vi "AlliGator Compute Phasor Plot Parameter Array.vi"(4 "Time Series Timestamps":dbl[](array[numeric]), 6 "Phasor Frequency":dbl[unit], 8 "error in (no error)":errorcluster, 9 "Parameter":T12=enum."Phasor g", 10 "Phasor Plot":T13, 11 "Raw Phasor Plot":T1 {"[Decay Metadata]"."# Folds" min=1; "[Decay Metadata]"."ROI Descriptor"."Contours"."Type" items=["No Selection", "Point", "Line", "Rectangle", "Oval", "Polygon", "Freehand Region", "Annulus", "Unused2", "Unused3", "Broken Line", "Freehand Line", "Rotated Rectangle"]}) -> (0 "error out":errorcluster, 3 "Parameter Array":dbl[](array[numeric]))   [LabVIEW 2021, in "AlliGator Phasor Graph.lvlib"]
doc: "Computes selected parameter for the phasors in a Phasor Plot of the Phasor Graph."
uses:
  AlliGator Phasor Graph.lvlib
  Graphs/XY Graph/XY Plot Data.ctl
  AlliGator Phasor Graph Parameter List.ctl
  AlliGator Raw Phasor Plot Data v4.ctl
  Phasor/Phasor (g, s).ctl
  AlliGator Decay Metadata v3.ctl
  AlliGator Decay Background Subtraction Info.ctl
  AlliGator Baseline Subtraction Method.ctl
  Graphs/XY Graph/XY Graph Plot Shift Parameters.ctl
  Graphs/XY Graph/XY Graph Plot Shift Method.ctl
  AlliGator Decay Extrapolation Parameters.ctl
  Phasor/Phasor Standard Deviation Options.ctl
  Phasor/Calibration Phasor (m, phi).ctl
  <userlib>/_OpenG.lib/array/array.llb/Filter 1D Array with Scalar (DBL)__ogtk.vi
  <userlib>/_OpenG.lib/array/array.llb/Delete Elements from 1D Array (Variant)__ogtk.vi
  <userlib>/_OpenG.lib/array/array.llb/Delete Elements from 1D Array (DBL)__ogtk.vi
  Phasor/Phasor.lvlib
  Image/Image.lvlib
  AlliGator Phasor Ratio.lvlib
  <userlib>/_OpenG.lib/array/array.llb/openg_array.lvlib
  Graphs/XY Graph/XY Graph Add-Ons.lvlib
  AlliGator Decay Preprocessing.lvlib
panel:
  # "see the AlliGator License on the block diagram (Ctrl+E or Window:Show Block Diagram)"
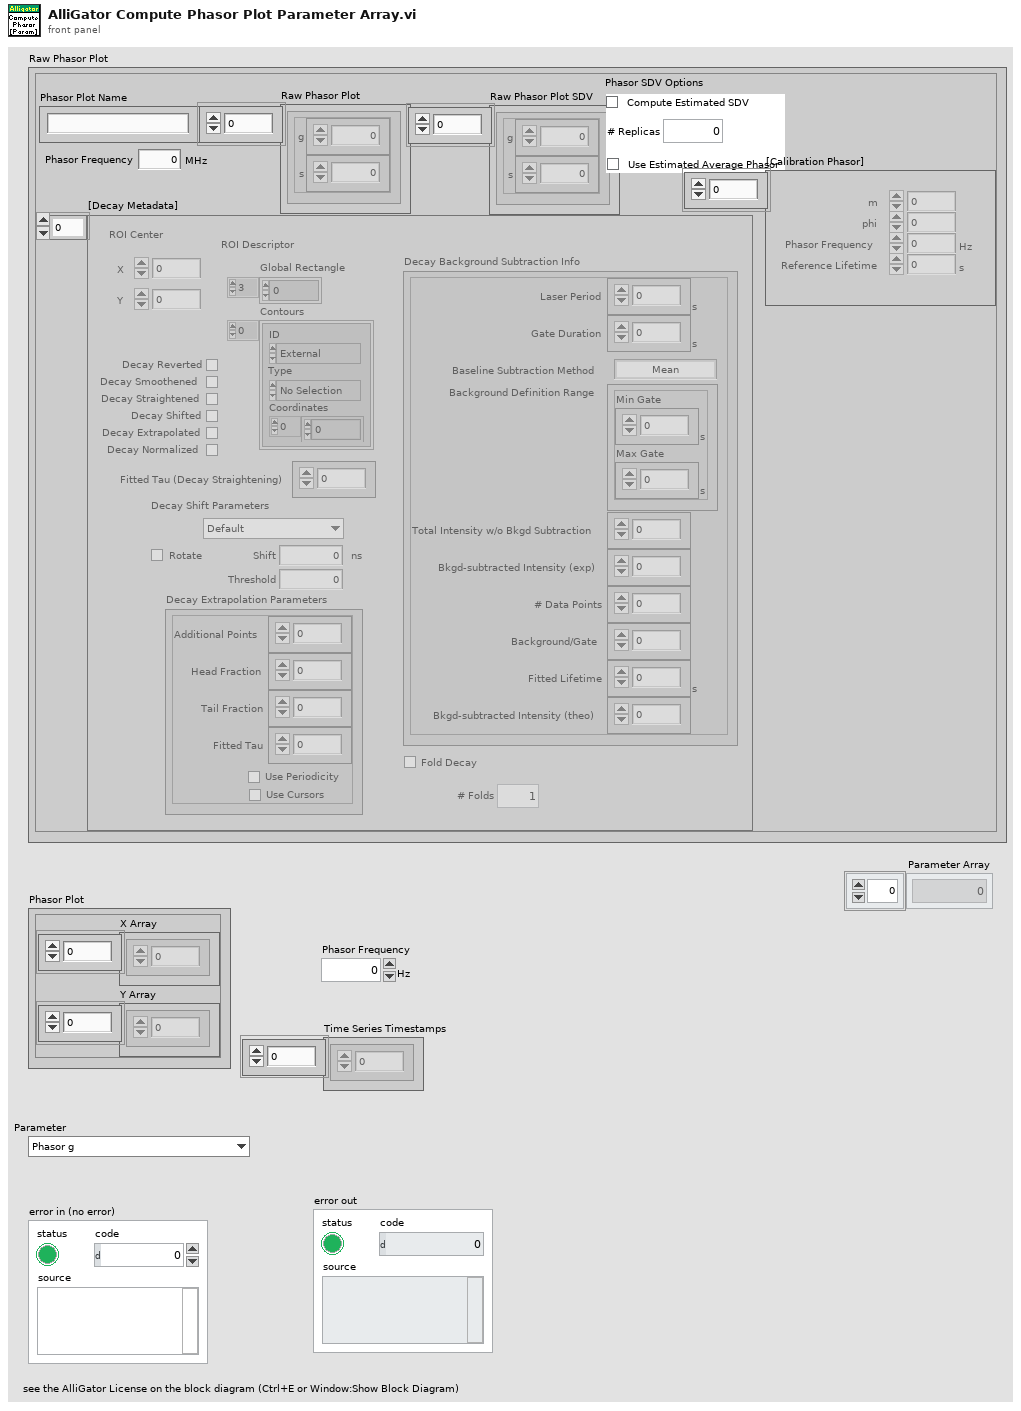
[diagram p1: front panel]
types:
  T1 = typedef "AlliGator Phasor Graph.lvlib/AlliGator Raw Phasor Plot Data v4.ctl" = cluster{"Phasor Plot Name":string, "Raw Phasor Plot":T2[], "Phasor Frequency":dbl[unit], "[Decay Metadata]":T3[], "Raw Phasor Plot SDV":T2[], "Phasor SDV Options":T10, "[Calibration Phasor]":T11[]}
  T2 = typedef "Phasor.lvlib/Phasor (g, s).ctl" = cluster{"g":dbl, "s":dbl}
  T3 = typedef "AlliGator Phasor Graph.lvlib/AlliGator Decay Metadata v3.ctl" = cluster{"ROI Descriptor":T4, "ROI Center":cluster{"X":i32, "Y":i32}, "Decay Background Subtraction Info":T5, "Decay Reverted":bool, "Decay Smoothened":bool, "Decay Straightened":bool, "Fitted Tau (Decay Straightening)":dbl, "Decay Shift Parameters":T7, "Decay Shifted":bool, "Decay Extrapolated":bool, "Decay Extrapolation Parameters":T9, "Decay Normalized":bool, "Fold Decay":bool, "# Folds":u32}
  T4 = typedef "ROI Descriptor" = cluster{"Global Rectangle":i32[], "Contours":cluster{"ID":enum32{"External", "Internal"}, "Type":u32, "Coordinates":i32[]}[]}
  T5 = typedef "AlliGator Decay Analysis.lvlib/AlliGator Decay Preprocessing.lvlib/AlliGator Decay Background Subtraction Info.ctl" = cluster{"Laser Period":dbl[unit], "Gate Duration":dbl[unit], "Baseline Subtraction Method":T6, "Background Definition Range":cluster{"Min Gate":dbl[unit], "Max Gate":dbl[unit]}, "Total Intensity w/o Bkgd Subtraction":dbl, "Bkgd-subtracted Intensity (exp)":dbl, "# Data Points":i32, "Background/Gate":dbl, "Fitted Lifetime":dbl[unit], "Bkgd-subtracted Intensity (theo)":dbl}
  T6 = typedef "AlliGator Decay Analysis.lvlib/AlliGator Decay Preprocessing.lvlib/AlliGator Baseline Subtraction Method.ctl" = enum16{"Mean", "Min", "Square Gated Single-Exponential", "File", "Constant"}
  T7 = typedef "XY Graph Add-Ons.lvlib/XY Graph Plot Shift Parameters.ctl" = cluster{"Type":T8, "Shift":dbl[unit], "Threshold":dbl, "Rotate":bool}
  T8 = typedef "XY Graph Add-Ons.lvlib/XY Graph Plot Shift Method.ctl" = enum16{"Default", "CFD", "Threshold", "Cross-Correlation"}
  T9 = typedef "AlliGator Decay Analysis.lvlib/AlliGator Decay Preprocessing.lvlib/AlliGator Decay Extrapolation Parameters.ctl" = cluster{"Additional Points":u32, "Head Fraction":dbl, "Fitted Tau":dbl, "Use Periodicity":bool, "Use Cursors":bool, "Tail Fraction":dbl}
  T10 = typedef "Phasor.lvlib/Phasor Standard Deviation Options.ctl" = cluster{"Compute Estimated SDV":bool, "# Replicas":u32, "Use Estimated Average Phasor":bool}
  T11 = typedef "Phasor.lvlib/Calibration Phasor (m, phi).ctl" = cluster{"m":dbl, "phi":dbl, "Phasor Frequency":dbl[unit], "Reference Lifetime":dbl[unit]}
  T12 = typedef "AlliGator Phasor Graph.lvlib/AlliGator Phasor Graph Parameter List.ctl" = enum16{"Time Stamp", "Index", "Phasor Parameters", "Phasor g", "Phasor s", "Phasor phi", "Phasor m", "Modulus Lifetime", "Phase Lifetime", "ROI Parameters", "ROI Center x", "ROI Center y", "ROI # pixels ", "Decay Parameters", "Intensity", "Background/Gate", "Intensity - Background", "Fitted Lifetime", "Fitted Intensity", "Phasor Ratio Parameters", "Amplitude Phasor Ratio", "Intensity Phasor Ratio", "Amplitude-Averaged Lifetime", "Intensity-Averaged Lifetime", "-", "Phasor Parameters SDV", "Phasor g SDV", "Phasor s SDV", "Phasor phi SDV", "Phasor m SDV", "Phase Lifetime SDV", "Modulus Lifetime SDV", "Phasor Ratio Parameters SDV", "Amplitude Phasor Ratio SDV", "Intensity Phasor Ratio SDV", "Amplitude-Averaged Lifetime SDV", "Intensity-Averaged Lifetime SDV"}
  T13 = typedef "XY Graph Add-Ons.lvlib/XY Plot Data.ctl" = cluster{"X Array":dbl[], "Y Array":dbl[]}
  T14 = typedef "Phasor.lvlib/Phasor (m, phi).ctl" = cluster{"m":dbl, "phi":dbl}
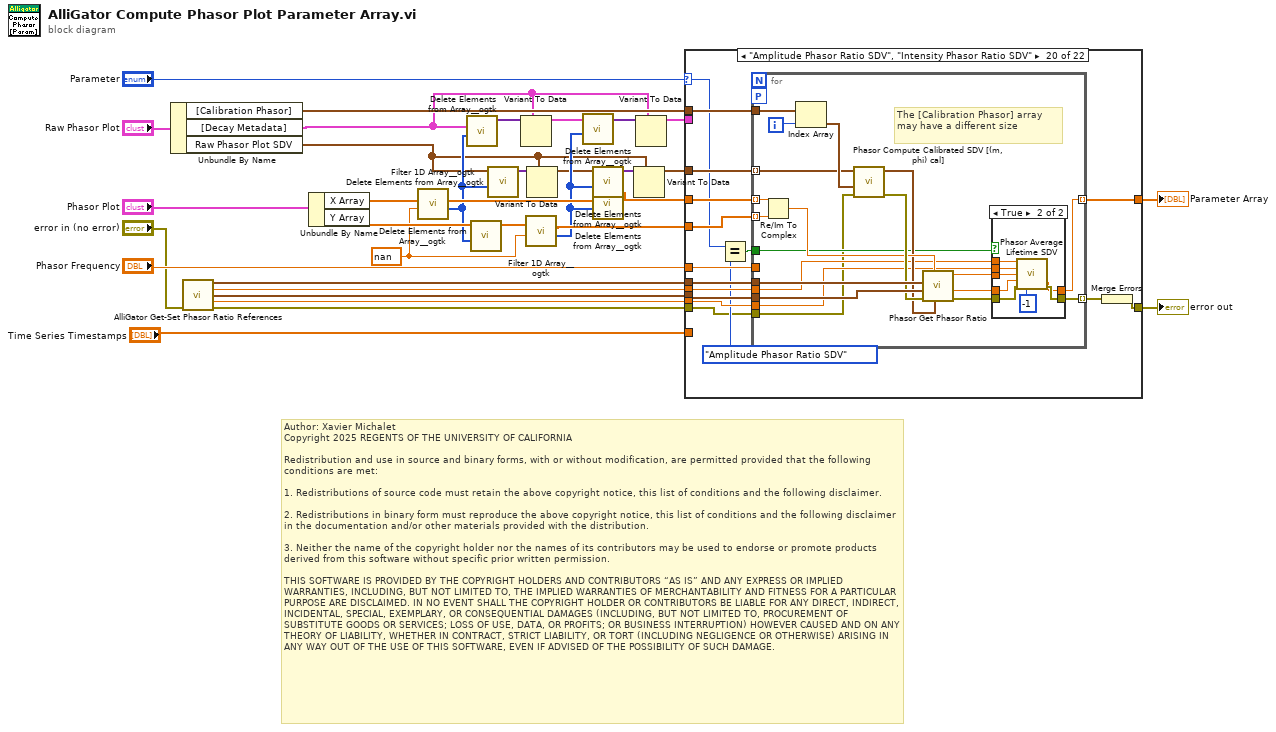
[diagram p0: block diagram]
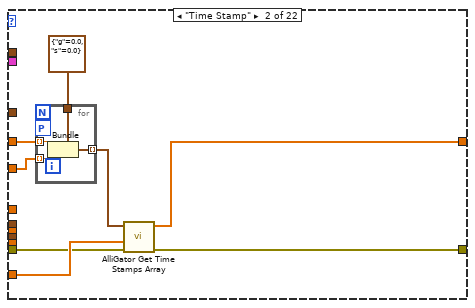
[diagram p3: hidden frame]
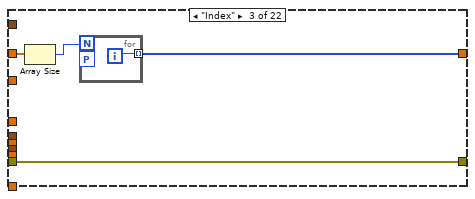
[diagram p4: hidden frame]
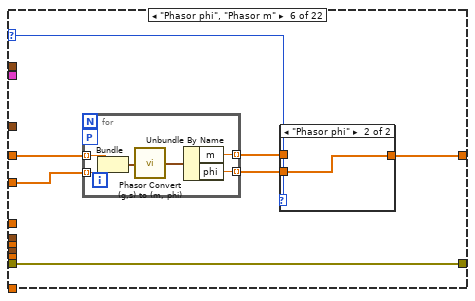
[diagram p7: hidden frame]
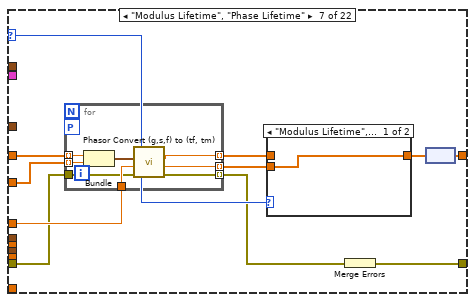
[diagram p9: hidden frame]
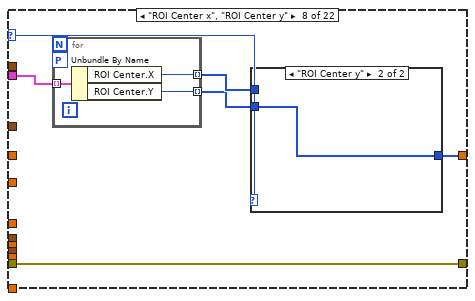
[diagram p11: hidden frame]
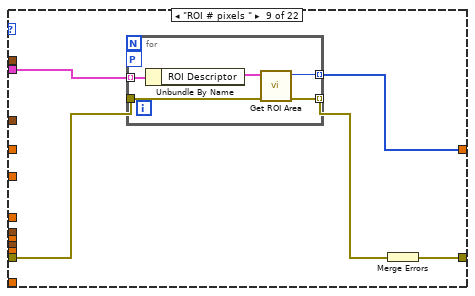
[diagram p13: hidden frame]
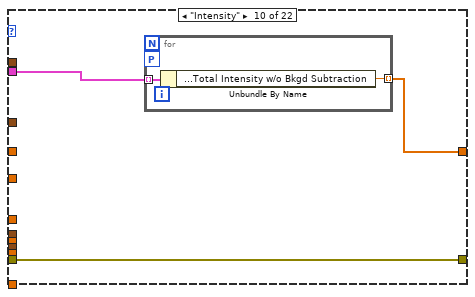
[diagram p14: hidden frame]
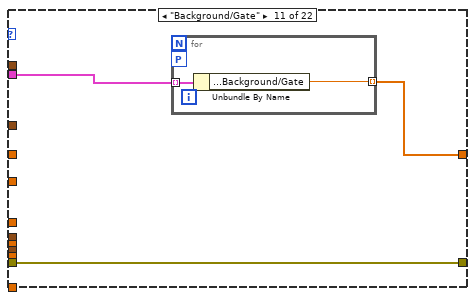
[diagram p15: hidden frame]
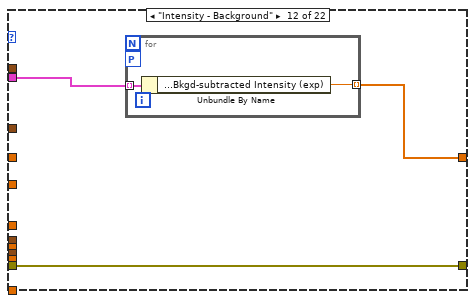
[diagram p16: hidden frame]
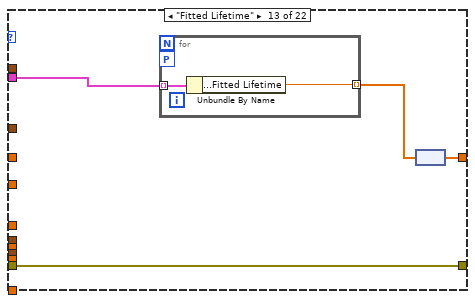
[diagram p17: hidden frame]
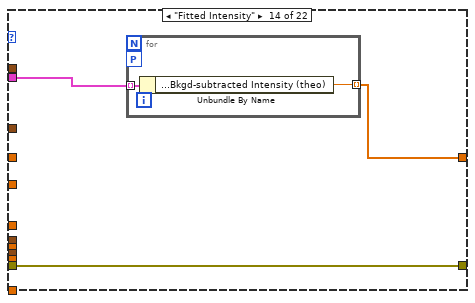
[diagram p18: hidden frame]
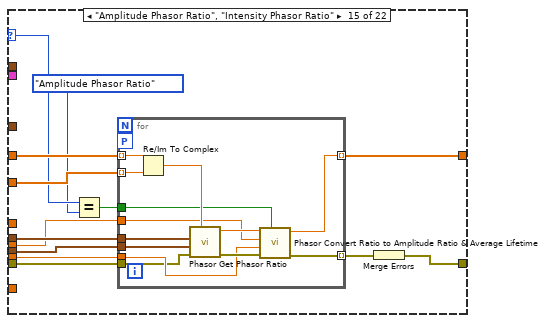
[diagram p19: hidden frame]
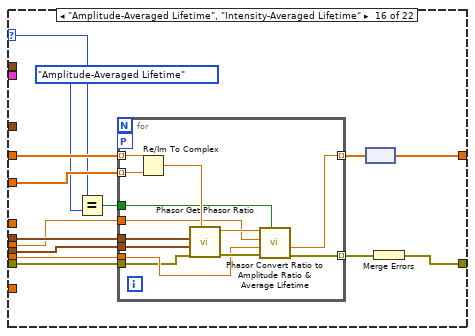
[diagram p20: hidden frame]
diagram:
  w14 = nan ("Numeric Control")
  # "Author: Xavier Michalet\nCopyright 2025 REGENTS OF THE UNIVERSITY OF CALIFORNIA\n\nRedistribution and use in source and binary forms, with or without modification, are permitted provided that the following conditions are met:\n\n1. Redistributions of source code must retain the above copyright notice, this list of conditions and the following disclaimer.\n\n2. Redistributions in binary form must reproduce the above copyright notice, this list of conditions and the following disclaimer in the documentation and/or other materials provided with the distribution.\n\n3. Neither the name of the copyright holder nor the names of its contributors may be used to endorse or promote products derived from this software without specific prior written permission.\n\nTHIS SOFTWARE IS PROVIDED BY THE COPYRIGHT HOLDERS AND CONTRIBUTORS “AS IS” AND ANY EXPRESS OR IMPLIED WARRANTIES, INCLUDING, BUT NOT LIMITED TO, THE IMPLIED WARRANTIES OF MERCHANTABILITY AND FITNESS FOR A PARTICULAR PURPOSE ARE DISCLAIMED. IN NO EVENT SHALL THE COPYRIGHT HOLDER OR CONTRIBUTORS BE LIABLE FOR ANY DIRECT, INDIRECT, INCIDENTAL, SPECIAL, EXEMPLARY, OR CONSEQUENTIAL DAMAGES (INCLUDING, BUT NOT LIMITED TO, PROCUREMENT OF SUBSTITUTE GOODS OR SERVICES; LOSS OF USE, DATA, OR PROFITS; OR BUSINESS INTERRUPTION) HOWEVER CAUSED AND ON ANY THEORY OF LIABILITY, WHETHER IN CONTRACT, STRICT LIABILITY, OR TORT (INCLUDING NEGLIGENCE OR OTHERWISE) ARISING IN ANY WAY OUT OF THE USE OF THIS SOFTWARE, EVEN IF ADVISED OF THE POSSIBILITY OF SUCH DAMAGE."
  n1 = Unbundle By Name("Raw Phasor Plot") -> ("[Calibration Phasor]"=w27:T11[], "[Decay Metadata]"=w4:T3[], "Raw Phasor Plot SDV"=w1:T2[])
  n2 = call "AlliGator Get-Set Phasor Ratio References.vi"("error in (no error)"="error in (no error)") -> ("Reference Phasor 1"=w30:T2, "Reference Lifetime 1"=w31:dbl[unit], "Reference Phasor 2"=w32:T2, "Reference Lifetime 2"=w33:dbl[unit], "error out"=w19:errorcluster)  [unwired: 7 in, 3 out]
  n3 = Unbundle By Name("Phasor Plot") -> ("X Array"=w29:dbl[], "Y Array"=w18:dbl[])
  n4 = call-poly <userlib>:"Filter 1D Array__ogtk.vi"("items to filter"=w14, "array"=w29) -> ("filtered item indices"=w11:i32[], "filtered array"=w13:dbl[])  [unwired: 4 in]
  n5 = call-poly <userlib>:"Delete Elements from Array__ogtk.vi"("indices"=w11, "array"=w4) -> ("array w/ subset deleted"=w16:variant[])  [unwired: 8 in, 1 out]
  n6 = call-poly <userlib>:"Delete Elements from Array__ogtk.vi"("indices"=w11, "array"=w18) -> ("array w/ subset deleted"=w17:dbl[])  [unwired: 8 in, 1 out]
  n7 = call-poly <userlib>:"Delete Elements from Array__ogtk.vi"("indices"=w11, "array"=w1) -> ("array w/ subset deleted"=w10:variant[])  [unwired: 8 in, 1 out]
  n8 = Variant To Data(type=w4, Variant=w16) -> (data=w8:T3[])  [unwired: 1 in, 1 out]
  n9 = call-poly <userlib>:"Filter 1D Array__ogtk.vi"("items to filter"=w14, "array"=w17) -> ("filtered item indices"=w9:i32[], "filtered array"=w15:dbl[])  [unwired: 4 in]
  n10 = Variant To Data(type=w1, Variant=w10) -> (data=w7:T2[])  [unwired: 1 in, 1 out]
  n11 = call-poly <userlib>:"Delete Elements from Array__ogtk.vi"("indices"=w9, "array"=w8) -> ("array w/ subset deleted"=w6:variant[])  [unwired: 8 in, 1 out]
  n12 = call-poly <userlib>:"Delete Elements from Array__ogtk.vi"("indices"=w9, "array"=w7) -> ("array w/ subset deleted"=w3:variant[])  [unwired: 8 in, 1 out]
  n13 = call-poly <userlib>:"Delete Elements from Array__ogtk.vi"("indices"=w9, "array"=w13) -> ("array w/ subset deleted"=w12:dbl[])  [unwired: 8 in, 1 out]
  n14 = Variant To Data(type=w1, Variant=w3) -> (data=w2:T2[])  [unwired: 1 in, 1 out]
  n15 = Variant To Data(type=w4, Variant=w6) -> (data=w5:T3[])  [unwired: 1 in, 1 out]
  n16 = case shown="\"Amplitude Phasor Ratio SDV\", \"Intensity Phasor Ratio SDV\"" "Parameter" {
    selector: "Parameter" -> [_ _ _ _ _ w60 w77 w97 _ _ _ _ _ _ w142 w168 w201 _ _ w263 w310 _]
    tunnel: w12 -> [_ w38 w50 w53 _ w62 w81 _ _ _ _ _ _ _ w149 w176 w196 w219 w241 w272 w319 _]
    tunnel: [_ w40 w49 w53 w55 w58 w79 w95 w107 w114 w119 w124 w129 w135 w143 w171 w199 w220 w242 w267 w307 _] -> w22
    tunnel: w15 -> [_ w37 _ _ w55 w61 w80 _ _ _ _ _ _ _ w148 w175 w195 w218 w240 w271 w318 _]
    tunnel: "Phasor Frequency" -> [_ _ _ _ _ _ w78 _ _ _ _ _ _ _ _ _ _ w221 w243 w273 w320 _]
    tunnel: w5 -> [_ _ _ _ _ _ _ w93 w106 w115 w120 w125 w131 w136 _ _ _ _ _ _ _ _]
    tunnel: w30 -> [_ _ _ _ _ _ _ _ _ _ _ _ _ _ w151 w178 _ _ _ w269 w316 _]
    tunnel: w31 -> [_ _ _ _ _ _ _ _ _ _ _ _ _ _ w146 w173 _ _ _ w265 w312 _]
    tunnel: w32 -> [_ _ _ _ _ _ _ _ _ _ _ _ _ _ w150 w177 _ _ _ w268 w315 _]
    tunnel: w33 -> [_ _ _ _ _ _ _ _ _ _ _ _ _ _ w147 w174 _ _ _ w264 w311 _]
    tunnel: w2 -> [_ _ _ _ _ _ _ _ _ _ _ _ _ _ _ _ w202 w215 w246 w275 w322 _]
    tunnel: [w34 w39 w48 w52 w54 w56 w72 w92 w103 w113 w118 w123 w128 w134 w144 w169 w193 w216 w238 w270 w317 w346] -> w25
    tunnel: w27 -> [_ _ _ _ _ _ _ _ _ _ _ _ _ _ _ _ w197 w223 w245 w274 w321 _]
    tunnel: w19 -> [w34 w41 w48 w52 w54 w56 w71 w92 w105 w113 w118 w123 w128 w134 w139 w165 w192 w214 w237 w260 w306 w346]
    tunnel: "Time Series Timestamps" -> [_ w42 _ _ _ _ _ _ _ _ _ _ _ _ _ _ _ _ _ _ _ _]
    frame "-", Default {
    }
    frame "Time Stamp" {
      n17 = for {
        tunnel: w38 -> [w46] mode=indexing
        tunnel: w37 -> [w45] mode=indexing
        tunnel: T2 {"g"=0.0, "s"=0.0} ("Phasor (g, s)") -> [w44]
        tunnel: [w43] -> w35 mode=indexing
        workers-P: _ -> [_]
        n18 = Bundle(cluster=w44, "g"=w46, "s"=w45) -> (w43:T2)
      }
      n19 = call "AlliGator Get Time Stamps Array.vi"("Error In"=w41, "Dataset Series Timestamps in"=w42, "Phasor Array"=w35) -> ("Error Out"=w39:errorcluster, "Dataset Series Timestamps out"=w40:dbl[])  [unwired: 7 in]
    }
    frame "Index" {
      n20 = Array Size(array=w50) -> (size(s)=w47:i32)
      n21 = for {
        N: w47 -> [_]
        tunnel: [w51] -> w49 mode=indexing
        workers-P: _ -> [_]
        i -> [w51]
      }
    }
    frame "Phasor g" {
    }
    frame "Phasor s" {
    }
    frame "Phasor phi", "Phasor m" {
      n22 = for {
        tunnel: w62 -> [w70] mode=indexing
        tunnel: w61 -> [w69] mode=indexing
        tunnel: [w66] -> w59 mode=indexing
        tunnel: [w65] -> w57 mode=indexing
        workers-P: _ -> [_]
        n23 = Bundle(w70, "Numeric"=w69) -> (w68:cluster{dbl, "Numeric":dbl})  [unwired: 1 in]
        n24 = call "Phasor Convert (g,s) to (m, phi).vi"("Phasor (g, s)"=w68) -> ("Phasor (m, phi)"=w67:T14)  [unwired: 8 in]
        n25 = Unbundle By Name(w67) -> ("m"=w66:dbl, "phi"=w65:dbl)
      }
      n26 = case shown="\"Phasor phi\"" w60 {
        tunnel: w59 -> [w63 _]
        tunnel: [w63 w64] -> w58
        tunnel: w57 -> [_ w64]
        frame "Phasor m", Default {
        }
        frame "Phasor phi" {
        }
      }
    }
    frame "Modulus Lifetime", "Phase Lifetime" {
      n27 = for {
        tunnel: w81 -> [w91] mode=indexing
        tunnel: w80 -> [w90] mode=indexing
        tunnel: [w88] -> w76 mode=indexing
        tunnel: [w87] -> w74 mode=indexing
        tunnel: w78 -> [w86]
        tunnel: [w85] -> w73 mode=indexing
        tunnel: w71 -> [w84]
        workers-P: _ -> [_]
        n28 = Bundle(w91, "Numeric"=w90) -> (w89:cluster{dbl, "Numeric":dbl})  [unwired: 1 in]
        n29 = call "Phasor Convert (g,s,f) to (tf, tm).vi"("Error In"=w84, "Phasor Harmonic Frequency"=w86, "Phasor (g, s)"=w89) -> ("Error Out"=w85:errorcluster, "Modulus Lifetime"=w87:dbl[unit], "Phase Lifetime"=w88:dbl[unit])  [unwired: 6 in]
      }
      n30 = case shown="\"Modulus Lifetime\", Default" w77 {
        tunnel: w76 -> [_ w83]
        tunnel: [w82 w83] -> w75
        tunnel: w74 -> [w82 _]
        frame "Modulus Lifetime", Default {
        }
        frame "Phase Lifetime" {
        }
      }
      n31 = Merge Errors(w73) -> (w72:errorcluster)
      n32 = node(w75) -> (w79:dbl[])
    }
    frame "ROI Center x", "ROI Center y" {
      n33 = for {
        tunnel: w93 -> [w102] mode=indexing
        tunnel: [w101] -> w96 mode=indexing
        tunnel: [w100] -> w94 mode=indexing
        workers-P: _ -> [_]
        n34 = Unbundle By Name(w102) -> ("ROI Center.X"=w101:i32, "ROI Center.Y"=w100:i32)
      }
      n35 = case shown="\"ROI Center y\"" w97 {
        tunnel: w96 -> [w98 _]
        tunnel: [w98 w99] -> w95
        tunnel: w94 -> [_ w99]
        frame "ROI Center x", Default {
        }
        frame "ROI Center y" {
        }
      }
    }
    frame "ROI # pixels " {
      n36 = for {
        tunnel: w106 -> [w112] mode=indexing
        tunnel: [w110] -> w107 mode=indexing
        tunnel: w105 -> [w109]
        tunnel: [w108] -> w104 mode=indexing
        workers-P: _ -> [_]
        n37 = Unbundle By Name(w112) -> ("ROI Descriptor"=w111:T4)
        n38 = call "Get ROI Area.vi"("Error In"=w109, "ROI Descriptor"=w111) -> ("Error Out"=w108:errorcluster, "Number of Pixels"=w110:u32)  [unwired: 8 in]
      }
      n39 = Merge Errors(w104) -> (w103:errorcluster)
    }
    frame "Intensity" {
      n40 = for {
        tunnel: w115 -> [w117] mode=indexing
        tunnel: [w116] -> w114 mode=indexing
        workers-P: _ -> [_]
        n41 = Unbundle By Name(w117) -> ("Decay Background Subtraction Info.Total Intensity w/o Bkgd Subtraction"=w116:dbl)
      }
    }
    frame "Background/Gate" {
      n42 = for {
        tunnel: w120 -> [w122] mode=indexing
        tunnel: [w121] -> w119 mode=indexing
        workers-P: _ -> [_]
        n43 = Unbundle By Name(w122) -> ("Decay Background Subtraction Info.Background/Gate"=w121:dbl)
      }
    }
    frame "Intensity - Background" {
      n44 = for {
        tunnel: w125 -> [w127] mode=indexing
        tunnel: [w126] -> w124 mode=indexing
        workers-P: _ -> [_]
        n45 = Unbundle By Name(w127) -> ("Decay Background Subtraction Info.Bkgd-subtracted Intensity (exp)"=w126:dbl)
      }
    }
    frame "Fitted Lifetime" {
      n46 = for {
        tunnel: w131 -> [w133] mode=indexing
        tunnel: [w132] -> w130 mode=indexing
        workers-P: _ -> [_]
        n47 = Unbundle By Name(w133) -> ("Decay Background Subtraction Info.Fitted Lifetime"=w132:dbl[unit])
      }
      n48 = node(w130) -> (w129:dbl[])
    }
    frame "Fitted Intensity" {
      n49 = for {
        tunnel: w136 -> [w138] mode=indexing
        tunnel: [w137] -> w135 mode=indexing
        workers-P: _ -> [_]
        n50 = Unbundle By Name(w138) -> ("Decay Background Subtraction Info.Bkgd-subtracted Intensity (theo)"=w137:dbl)
      }
    }
    frame "Amplitude Phasor Ratio", "Intensity Phasor Ratio" {
      n51 = Equal?(x=w142, y=AlliGator_Phasor_Graph_Parameter_List."Amplitude Phasor Ratio") -> (x = y?=w141:bool)
      n52 = for {
        tunnel: w151 -> [w164]
        tunnel: w150 -> [w163]
        tunnel: w149 -> [w162] mode=indexing
        tunnel: w148 -> [w161] mode=indexing
        tunnel: w147 -> [w157]
        tunnel: w146 -> [w156]
        tunnel: [w154] -> w143 mode=indexing
        tunnel: [w155] -> w145 mode=indexing
        tunnel: w141 -> [w153]
        tunnel: w139 -> [w152]
        workers-P: _ -> [_]
        n53 = Re/Im To Complex(1:w161, 2:w162) -> (0:w160:cdb)
        n54 = call "Phasor Get Phasor Ratio.vi"("z"=w160, "Error In"=w152, "Reference Phasor 2"=w163, "Reference Phasor 1"=w164) -> ("Error Out"=w158:errorcluster, "Phasor Ratio (f1)"=w159:dbl)  [unwired: 5 in, 1 out]
        n55 = call "Phasor Convert Ratio to Amplitude Ratio & Average Lifetime.vi"("Compute Amplitude Ratio"=w153, "error in (no error)"=w158, "Reference Lifetime 2"=w157, "Reference Lifetime 1"=w156, "Phasor Ratio (f1)"=w159) -> ("error out"=w155:errorcluster, "Phasor/Amplitude Ratio"=w154:dbl)  [unwired: 2 in, 3 out]
      }
      n56 = Merge Errors(w145) -> (w144:errorcluster)
    }
    frame "Amplitude-Averaged Lifetime", "Intensity-Averaged Lifetime" {
      n57 = Equal?(x=w168, y=AlliGator_Phasor_Graph_Parameter_List."Amplitude-Averaged Lifetime") -> (x = y?=w167:bool)
      n58 = for {
        tunnel: w178 -> [w191]
        tunnel: w177 -> [w190]
        tunnel: w176 -> [w189] mode=indexing
        tunnel: w175 -> [w188] mode=indexing
        tunnel: w174 -> [w184]
        tunnel: w173 -> [w183]
        tunnel: [w182] -> w172 mode=indexing
        tunnel: [w181] -> w170 mode=indexing
        tunnel: w167 -> [w180]
        tunnel: w165 -> [w179]
        workers-P: _ -> [_]
        n59 = Re/Im To Complex(1:w188, 2:w189) -> (0:w187:cdb)
        n60 = call "Phasor Get Phasor Ratio.vi"("z"=w187, "Error In"=w179, "Reference Phasor 2"=w190, "Reference Phasor 1"=w191) -> ("Error Out"=w185:errorcluster, "Phasor Ratio (f1)"=w186:dbl)  [unwired: 5 in, 1 out]
        n61 = call "Phasor Convert Ratio to Amplitude Ratio & Average Lifetime.vi"("Compute Amplitude Ratio"=w180, "error in (no error)"=w185, "Reference Lifetime 2"=w184, "Reference Lifetime 1"=w183, "Phasor Ratio (f1)"=w186) -> ("error out"=w181:errorcluster, "Average Lifetime"=w182:dbl[unit])  [unwired: 2 in, 3 out]
      }
      n62 = node(w172) -> (w171:dbl[])
      n63 = Merge Errors(w170) -> (w169:errorcluster)
    }
    frame "Phasor g SDV", "Phasor s SDV" {
      # "The [Calibration Phasor] array may have a different size"
      n64 = for {
        tunnel: w202 -> [w206] mode=indexing
        tunnel: [w213] -> w200 mode=indexing
        tunnel: [w212] -> w198 mode=indexing
        tunnel: w197 -> [w211]
        tunnel: w196 -> [_] mode=indexing
        tunnel: w195 -> [_] mode=indexing
        tunnel: [w207] -> w194 mode=indexing
        tunnel: w192 -> [w205]
        workers-P: _ -> [_]
        i -> [w210]
        n65 = Index Array(array=w211, index=w210) -> (element=w209:T11)
        n66 = call "Phasor Compute Calibrated SDV [(m, phi) cal].vi"("error in"=w205, "Calibration Phasor"=w209, "Raw Phasor"=w206) -> ("error out"=w207:errorcluster, "Calibrated Phasor SDV (g, s)"=w208:T2)  [unwired: 7 in]
        n67 = Unbundle By Name(w208) -> ("g"=w213:dbl, "s"=w212:dbl)
      }
      n68 = case shown="\"Phasor s\"" w201 {
        tunnel: w200 -> [w203 _]
        tunnel: [w203 w204] -> w199
        tunnel: w198 -> [_ w204]
        frame "Phasor g", Default {
        }
        frame "Phasor s" {
        }
      }
      n69 = Merge Errors(w194) -> (w193:errorcluster)
    }
    frame "Phase Lifetime SDV" {
      # "The [Calibration Phasor] array may have a different size"
      n70 = for {
        tunnel: [w234] -> w222 mode=indexing
        tunnel: w223 -> [w236]
        tunnel: w221 -> [w233]
        tunnel: w219 -> [w232] mode=indexing
        tunnel: w218 -> [w231] mode=indexing
        tunnel: [w230] -> w217 mode=indexing
        tunnel: w215 -> [w225] mode=indexing
        tunnel: w214 -> [w224]
        workers-P: _ -> [_]
        i -> [w235]
        n71 = Bundle(w232, "Numeric"=w231) -> (w226:cluster{dbl, "Numeric":dbl})  [unwired: 1 in]
        n72 = Index Array(array=w236, index=w235) -> (element=w229:T11)
        n73 = call "Phasor Compute Calibrated SDV [(m, phi) cal].vi"("error in"=w224, "Calibration Phasor"=w229, "Raw Phasor"=w225) -> ("error out"=w228:errorcluster, "Calibrated Phasor SDV (g, s)"=w227:T2)  [unwired: 7 in]
        n74 = call "Phasor Compute tau_phi SDV.vi"("Error In"=w228, "Phasor Frequency"=w233, "Phasor SDV (g, s)"=w227, "Phasor (g, s)"=w226) -> ("Error Out"=w230:errorcluster, "tau_phi SDV"=w234:dbl[unit])  [unwired: 6 in]
      }
      n75 = Merge Errors(w217) -> (w216:errorcluster)
      n76 = node(w222) -> (w220:dbl[])
    }
    frame "Modulus Lifetime SDV" {
      # "The [Calibration Phasor] array may have a different size"
      n77 = for {
        tunnel: w246 -> [w248] mode=indexing
        tunnel: [w257] -> w244 mode=indexing
        tunnel: w245 -> [w259]
        tunnel: w243 -> [w256]
        tunnel: w241 -> [w253] mode=indexing
        tunnel: w240 -> [w252] mode=indexing
        tunnel: [w251] -> w239 mode=indexing
        tunnel: w237 -> [w247]
        workers-P: _ -> [_]
        i -> [w258]
        n78 = Bundle(w253, "Numeric"=w252) -> (w250:cluster{dbl, "Numeric":dbl})  [unwired: 1 in]
        n79 = Index Array(array=w259, index=w258) -> (element=w249:T11)
        n80 = call "Phasor Compute Calibrated SDV [(m, phi) cal].vi"("error in"=w247, "Calibration Phasor"=w249, "Raw Phasor"=w248) -> ("error out"=w255:errorcluster, "Calibrated Phasor SDV (g, s)"=w254:T2)  [unwired: 7 in]
        n81 = call "Phasor Compute tau_m SDV.vi"("Error In"=w255, "Phasor Frequency"=w256, "Phasor SDV (g, s)"=w254, "Phasor (g, s)"=w250) -> ("Error Out"=w251:errorcluster, "<tau_m>"=w257:dbl[unit])  [unwired: 5 in, 1 out]
      }
      n82 = Merge Errors(w239) -> (w238:errorcluster)
      n83 = node(w244) -> (w242:dbl[])
    }
    frame "Amplitude Phasor Ratio SDV", "Intensity Phasor Ratio SDV" {
      n84 = Equal?(x=w263, y=AlliGator_Phasor_Graph_Parameter_List."Amplitude Phasor Ratio SDV") -> (x = y?=w261:bool)
      n85 = for {
        tunnel: w275 -> [w289] mode=indexing
        tunnel: w274 -> [w295]
        tunnel: w273 -> [_]
        tunnel: w272 -> [w288] mode=indexing
        tunnel: w271 -> [w287] mode=indexing
        tunnel: w269 -> [w293]
        tunnel: w268 -> [w292]
        tunnel: [w277] -> w267 mode=indexing
        tunnel: [w278] -> w266 mode=indexing
        tunnel: w265 -> [w281]
        tunnel: w264 -> [w280]
        tunnel: w261 -> [w279]
        tunnel: w260 -> [w276]
        workers-P: _ -> [_]
        i -> [w294]
        # "The [Calibration Phasor] array may have a different size"
        n86 = Re/Im To Complex(1:w287, 2:w288) -> (0:w286:cdb)
        n87 = Index Array(array=w295, index=w294) -> (element=w291:T11)
        n88 = call "Phasor Compute Calibrated SDV [(m, phi) cal].vi"("error in"=w276, "Calibration Phasor"=w291, "Raw Phasor"=w289) -> ("error out"=w290:errorcluster, "Calibrated Phasor SDV (g, s)"=w285:T2)  [unwired: 7 in]
        n89 = call "Phasor Get Phasor Ratio.vi"("Phasor SDV"=w285, "z"=w286, "Error In"=w290, "Reference Phasor 2"=w292, "Reference Phasor 1"=w293) -> ("Error Out"=w282:errorcluster, "Phasor Ratio SDV"=w283:dbl, "Phasor Ratio (f1)"=w284:dbl)  [unwired: 4 in]
        n90 = case shown="True" w279 {
          tunnel: w284 -> [_ w305]
          tunnel: w283 -> [w296 w304]
          tunnel: w282 -> [w297 w303]
          tunnel: w281 -> [_ w302]
          tunnel: w280 -> [_ w301]
          tunnel: [w297 w300] -> w278
          tunnel: [w296 w299] -> w277
          frame False {
          }
          frame True {
            n91 = call "Phasor Average Lifetime SDV.vi"("tau 1"=w302, "tau 2"=w301, "r"=w305, "SDV r"=w304, "Error In"=w303, "seed"=-1) -> ("SDV a"=w299:dbl, "Error Out"=w300:errorcluster)  [unwired: 4 in, 4 out]
          }
        }
      }
      n92 = Merge Errors(w266) -> (w270:errorcluster)
    }
    frame "Amplitude-Averaged Lifetime SDV", "Intensity-Averaged Lifetime SDV" {
      n93 = Equal?(x=w310, y=AlliGator_Phasor_Graph_Parameter_List."Amplitude Phasor Ratio SDV") -> (x = y?=w308:bool)
      n94 = for {
        tunnel: w322 -> [w339] mode=indexing
        tunnel: w321 -> [w345]
        tunnel: w320 -> [_]
        tunnel: w319 -> [w338] mode=indexing
        tunnel: w318 -> [w337] mode=indexing
        tunnel: w316 -> [w343]
        tunnel: w315 -> [w342]
        tunnel: [w325] -> w314 mode=indexing
        tunnel: [w329] -> w313 mode=indexing
        tunnel: w312 -> [w331]
        tunnel: w311 -> [w330]
        tunnel: w308 -> [w328]
        tunnel: w306 -> [w324]
        workers-P: _ -> [_]
        i -> [w344]
        # "The [Calibration Phasor] array may have a different size"
        n95 = Re/Im To Complex(1:w337, 2:w338) -> (0:w336:cdb)
        n96 = Index Array(array=w345, index=w344) -> (element=w341:T11)
        n97 = call "Phasor Compute Calibrated SDV [(m, phi) cal].vi"("error in"=w324, "Calibration Phasor"=w341, "Raw Phasor"=w339) -> ("error out"=w340:errorcluster, "Calibrated Phasor SDV (g, s)"=w335:T2)  [unwired: 7 in]
        n98 = call "Phasor Get Phasor Ratio.vi"("Phasor SDV"=w335, "z"=w336, "Error In"=w340, "Reference Phasor 2"=w342, "Reference Phasor 1"=w343) -> ("Error Out"=w332:errorcluster, "Phasor Ratio SDV"=w333:dbl, "Phasor Ratio (f1)"=w334:dbl)  [unwired: 4 in]
        n99 = call "Phasor Average Lifetime SDV.vi"("tau 1"=w331, "tau 2"=w330, "r"=w334, "SDV r"=w333, "Error In"=w332, "seed"=-1) -> ("SDV <tau>_a"=w327:dbl[unit], "SDV <tau>_i"=w326:dbl[unit], "Error Out"=w329:errorcluster)  [unwired: 4 in, 3 out]
        n100 = Select(t=w327, s=w328, f=w326) -> (s? t:f=w325:dbl[unit])
      }
      n101 = node(w314) -> (w307:dbl[])
      n102 = Merge Errors(w313) -> (w317:errorcluster)
    }
    frame "Phasor phi SDV", "Phasor m SDV" {
      # "Not supported"
      # "The [Calibration Phasor] array may have a different size"
    }
  }
  "error out" <- w25
  "Parameter Array" <- w22
